vi "Import Export - Export to XML File.vi"(8 "error in":errorcluster, 10 "Configuration File Path":path, 11 "Item Ref in":T1 format="%.0x") -> (0 "error out":errorcluster, 3 "Item Ref out":T1 format="%.0x", 4 "xml string":string)   [LabVIEW 2017, in "PXImc System Explorer.lvlib"]
uses:
  PXImc System Explorer.lvlib
  <vilib>/NI Veristand/Custom Device API/Custom Device Item Ref.ctl
  <vilib>/NI/NI VeriStand Custom Device Import and Export Tool/ImportExport.lvlib
  <vilib>/NI Veristand/Custom Device API/Custom Device API.lvlib
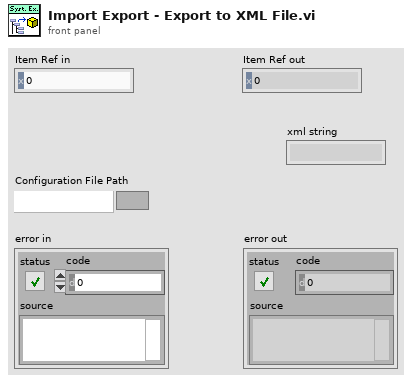
[diagram p1: front panel]
types:
  T1 = typedef "Custom Device API.lvlib/Custom Device Item Ref.ctl" = u64
  T2 = typedef "Advanced System Definition.lvlib/SysDef.Export.ctl" = cluster{"Version":string, "Tree":T3[]}
  T3 = typedef "Advanced System Definition.lvlib/TreeItem.ctl" = cluster{"Item Info":T4, "Parent Path":string[], "Properties":T9[]}
  T4 = typedef "Advanced System Definition.lvlib/TreeItem.Info.ctl" = cluster{"Name":string, "Description":string, "GUID":string, "Is Channel":bool, "Channel":T5, "Is Waveform":bool, "Waveform":T7}
  T5 = typedef "Custom Device API.lvlib/Custom Device Channel.ctl" = cluster{"Type":T6, "Units":string, "Default Value":dbl, "Faultable":bool, "Scalable":bool}
  T6 = typedef "Custom Device API.lvlib/Custom Device Channel Type.ctl" = enum16{"Input", "Output"}
  T7 = typedef "Custom Device API.lvlib/Custom Device Waveform.ctl" = cluster{"Data Type":T8, "Units":string}
  T8 = typedef "Custom Device API.lvlib/Custom Device Waveform DataType.ctl" = enum16{"Double", "Complex Double"}
  T9 = typedef "Advanced System Definition.lvlib/TreeItem.Property.ctl" = cluster{"Name":string, "Type":i32, "Value":variant}
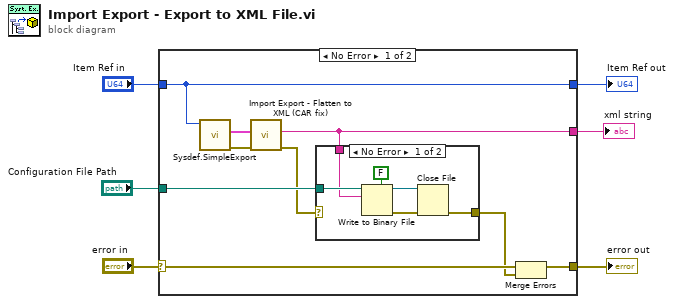
[diagram p0: block diagram]
diagram:
  n1 = case shown="No Error" "error in" {
    selector: "error in" -> [w15 w23]
    tunnel: [w12 w23] -> w5
    tunnel: [w14 w24] -> w4
    tunnel: "Item Ref in" -> [w14 w24]
    tunnel: "Configuration File Path" -> [w13 _]
    tunnel: [w10 _] -> w1
    frame No Error {
      n2 = call <vilib>:"Sysdef.SimpleExport.vi"("ID"=w14) -> ("error out"=w9:errorcluster, "Export"=w7:T2)  [unwired: 8 in, 1 out]
      n3 = call "Import Export - Flatten to XML (CAR fix).vi"("Error In"=w9, "Export"=w7) -> ("Error Out"=w8:errorcluster, "XML String Out"=w10:string)  [unwired: 8 in]
      n4 = case shown="No Error" w8 {
        selector: w8 -> [_ w22]
        tunnel: w13 -> [w18 _]
        tunnel: w10 -> [w16 _]
        tunnel: [w20 w22] -> w11
        frame No Error {
          n5 = Write to Binary File(file (use dialog)=w18, data=w16, 5:FALSE ("prepend array or string size? (T)")) -> (refnum out=w21:refnum<file>, error out=w19:errorcluster)  [unwired: 1 in, 3 out]
          n6 = Close File(refnum=w21, error in=w19) -> (error out=w20:errorcluster)  [unwired: 1 out]
        }
        frame Error {
        }
      }
      n7 = Merge Errors(w15, w11) -> (w12:errorcluster)
    }
    frame Error {
    }
  }
  "error out" <- w5
  "Item Ref out" <- w4
  "xml string" <- w1
